vi "Average Signal Voltage.vi"(2 "leading samples to kill (0)":i32, 3 "voltage data":dbl[][](array[numeric]) format="%.2f") -> (1 "average value\nper channel":dbl[](array[numeric]) format="%.2f")   [LabVIEW 2013]
doc: "Accepts raw 2D voltage array from a DAQ scan function and averages each channel's data into a single value. Deletes selected number of samples from the beginning of the data to get rid of settling time problems. Applies offset and scale calibration info from the configuration to produce results in engineering units. Output is an array with one value per channel, all single-precision."
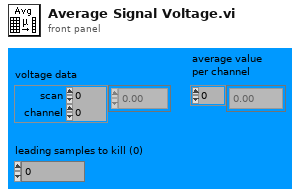
[diagram p1: front panel]
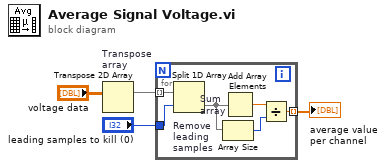
[diagram p0: block diagram]
diagram:
  n1 = Transpose 2D Array "Transpose\narray"(2D array="voltage data") -> (transposed array=w3:dbl[][])
  n2 = for {
    tunnel: w3 -> [w10] mode=indexing
    tunnel: "leading samples to kill (0)" -> [w9]
    tunnel: [w5] -> w1 mode=indexing
    n3 = Split 1D Array "Remove\nleading\nsamples"(array=w10, index=w9) -> (second subarray=w8:dbl[])  [unwired: 1 out]
    n4 = Array Size(array=w8) -> (size(s)=w6:i32)
    n5 = Add Array Elements "Sum\narray"(numeric array=w8) -> (sum=w7:dbl)
    n6 = Divide(x=w7, y=w6) -> (x/y=w5:dbl)
  }
  "average value\nper channel" <- w1
